vi "Get Result.vi"(8 "error in (no error)":errorcluster, 11 "Keithley Meter in":refnum<class "Keithley 182.lvclass">) -> (0 "error out":errorcluster, 2 "Mag Lab Result.lvclass":refnum<class "Mag Lab Result.lvclass">, 3 "Keithley Meter out":refnum<class "Keithley 182.lvclass">)   [LabVIEW 2015, in "Keithley 182.lvclass"]
uses:
  Keithley 182.lvclass
  Mag Lab Result/Mag Lab Result.lvclass
  Mag Lab Hardware.lvclass/Mag Lab Hardware.ctl
  Mag Lab Root/Mag Lab Root.lvclass/Mag Lab Root.ctl
  Mag Lab Hardware.lvclass
  Mag Lab Error Handler/Mag Lab Error Handler.lvclass
  Mag Lab Root/Mag Lab Root.lvclass
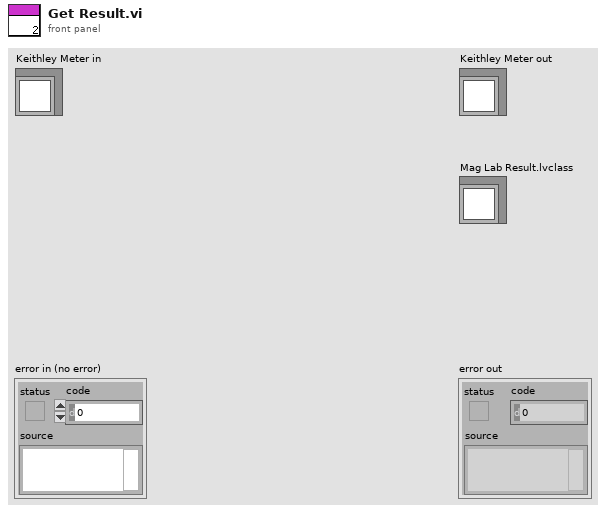
[diagram p1: front panel]
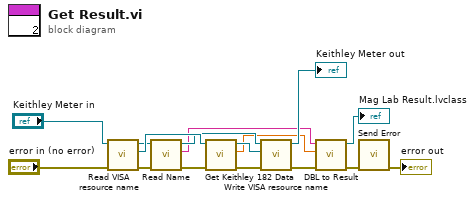
[diagram p0: block diagram]
diagram:
  n1 = call "Read VISA resource name.vi"("error in (no error)"="error in (no error)", "Mag Lab Hardware in"="Keithley Meter in") -> ("error out"=w13:errorcluster, "VISA resource name"=w15:refnum<visa-resource-name>, "Mag Lab Hardware out"=w14:refnum<class "Keithley 182.lvclass">)  [unwired: 7 in]
  n2 = call "Read Name.vi"("error in (no error)"=w13, "Mag Lab Root in"=w14) -> ("error out"=w12:errorcluster, "Name"=w5:string, "Mag Lab Root out"=w11:refnum<class "Keithley 182.lvclass">)  [unwired: 7 in]
  n3 = call "Get Keithley 182 Data.vi"("error in (no error)"=w12, "VISA Resource Name"=w15) -> ("error out"=w8:errorcluster, "Data"=w4:dbl, "VISA Resource Name Out"=w10:refnum<visa-resource-name>)  [unwired: 6 in, 1 out]
  n4 = call "Write VISA resource name.vi"("error in (no error)"=w8, "VISA resource name"=w10, "Mag Lab Hardware in"=w11) -> ("error out"=w2:errorcluster, "Mag Lab Hardware out"=→"Keithley Meter out":refnum<class "Keithley 182.lvclass">)  [unwired: 7 in]
  n5 = call "DBL to Result.vi"("error in (no error)"=w2, "Data"=w4, "Name"=w5) -> ("error out"=w1:errorcluster, "Mag Lab Result out"=→"Mag Lab Result.lvclass":refnum<class "Mag Lab Result.lvclass">)  [unwired: 7 in]
  n6 = call "Send Error.vi"("error in (no error)"=w1) -> ("error out"=→"error out":errorcluster)  [unwired: 9 in, 1 out]
